vi "yrescale.vi"(10 "scalingfactor":dbl, 11 "ylabview":dbl) -> (3 "function return":dbl)   [LabVIEW 2017, in "HapticSTM.lvlib"]
doc: "extern \"C\" __declspec(dllexport) double yrescale(double ylabview, double scalingfactor);"
uses:
  <userlib>/HapticSTM/Feedbackless - Testdata/Zthreshholdtesting 2017 version/Zthreshholdtestingtestytest/HapticSTM.lvlib
  <userlib>/HapticSTM/HapticSTM.dll
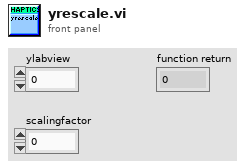
[diagram p1: front panel]
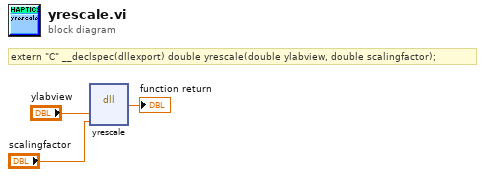
[diagram p0: block diagram]
diagram:
  # "extern \"C\" __declspec(dllexport) double yrescale(double ylabview, double scalingfactor);"
  n1 = dll-call lib="C:/Program Files/National Instruments/LabVIEW 2019/user.lib/HapticSTM/HapticSTM.*" fn="yrescale"("ylabview"="ylabview", "scalingfactor"="scalingfactor") -> (→"function return":dbl)  [unwired: 5 in, 2 out]
